vi "CoboltLaser_TECdrivesGet.vi"(0 "ComPort":refnum<visa-resource-name>, 3 "CheckResponse":bool=TRUE, 7 "error in (no error)":errorcluster) -> (20 "ComPortOut":refnum<visa-resource-name>, 21 "TEC drive":dbl[](array[numeric]), 27 "error out":errorcluster)   [LabVIEW 2012, in "Cobolt.lvclass"]
doc: "Use this template to build a VI to use as a subVI."
uses:
  Template/Cobolt.lvclass
panel:
  out "ResponseOK":bool
  out "Response":string
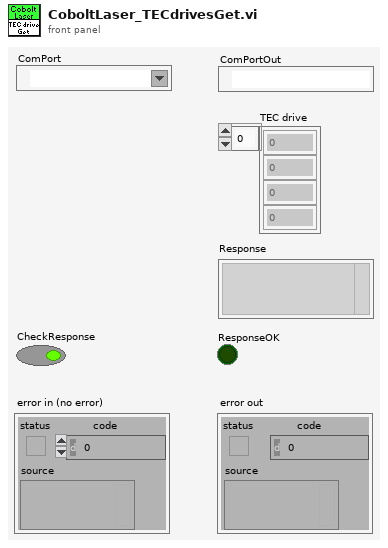
[diagram p1: front panel]
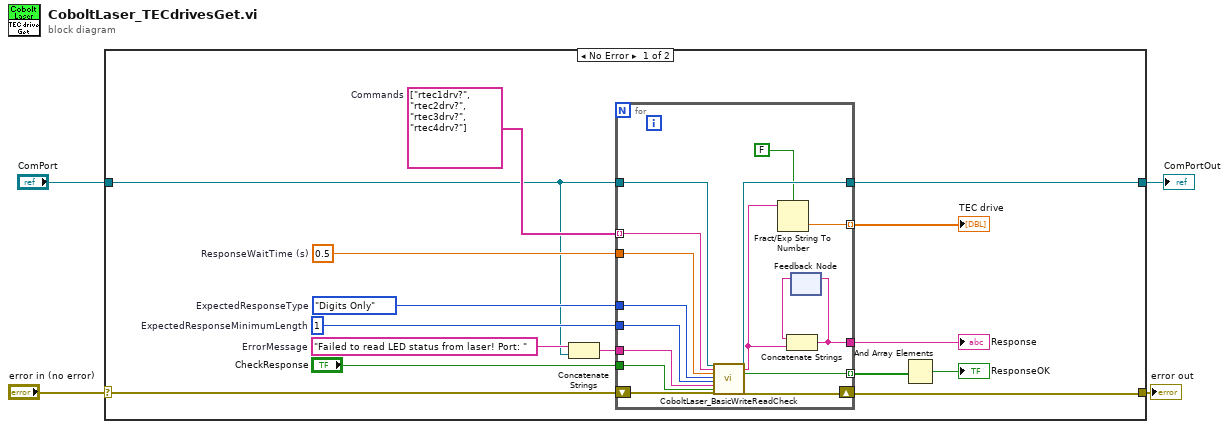
[diagram p0: block diagram]
diagram:
  n1 = case shown="No Error" "error in (no error)" {
    selector: "error in (no error)" -> [w19 w37]
    tunnel: [w18 w37] -> w3
    tunnel: "ComPort" -> [w6 w36]
    tunnel: [w5 w36] -> w1
    frame No Error {
      w11 = string[] ["rtec1drv?", "rtec2drv?", "rtec3drv?", "rtec4drv?"]  # Commands
      w15 = 1  # ExpectedResponseMinimumLength
      w16 = enum16{"Any", "Digits Only", "Non-Digits Only"}."Digits Only"  # ExpectedResponseType
      w17 = 0.5  # ResponseWaitTime (s)
      w13 = "Failed to read LED status from laser! Port: "  # ErrorMessage
      n2 = Concatenate Strings(w13, w6) -> (w12:string)
      n3 = for {
        tunnel: w17 -> [w33]
        tunnel: w11 -> [w32] mode=indexing
        tunnel: w16 -> [w31]
        tunnel: w15 -> [w30]
        tunnel: "CheckResponse" -> [w29]
        tunnel: [w28] -> w5
        tunnel: [w27] -> w10 mode=indexing
        tunnel: w12 -> [w26]
        tunnel: w6 -> [w25]
        shift-right: [w34] -> w18
        shift-left: w19 -> [w35]
        tunnel: [w24] -> w7 mode=indexing
        tunnel: [w21] -> w8
        n4 = call "CoboltLaser_BasicWriteReadCheck.vi"("ComPort"=w25, "Command"=w32, "ResponseWaitTime (s)"=w33, "ExpectedResponseType"=w31, "ExpectedResponseMinimumLength"=w30, "ErrorMessage"=w26, "CheckResponse"=w29, "error in (no error)"=w35) -> ("ComPortOut"=w28:refnum<visa-resource-name>, "Response"=w23:string, "ResponseOK"=w27:bool, "error out"=w34:errorcluster)  [unwired: 16 in]
        n5 = Fract/Exp String To Number(use system decimal point (T)=FALSE, string=w23) -> (number=w24:dbl)  [unwired: 2 in, 1 out]
        n6 = feedback #1() -> (w22:string)  [unwired: 1 in]
        n7 = Concatenate Strings(w22, w23) -> (w21:string)
        n8 = feedback-in #1(w21) -> ()
      }
      "Response" <- w8
      "TEC drive" <- w7
      n9 = And Array Elements(Boolean array=w10) -> (logical AND=→"ResponseOK":bool)
    }
    frame Error {
    }
  }
  "error out" <- w3
  "ComPortOut" <- w1
